vi "Update and Rename Files.vi"(8 "error in":errorcluster, 9 "Type ID":string="test", 10 "New Name":string="test", 11 "New PE Folder":path=path "C:/Users/carls/Desktop/test") -> (0 "error out":errorcluster)   [LabVIEW 2020, in "ADAS_IO_Template_MDO.lvclass"]
uses:
  ADAS_IO_Template_MDO.lvclass
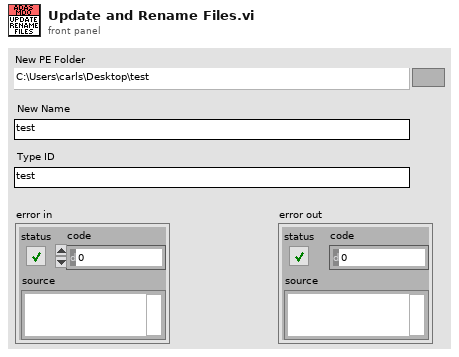
[diagram p1: front panel]
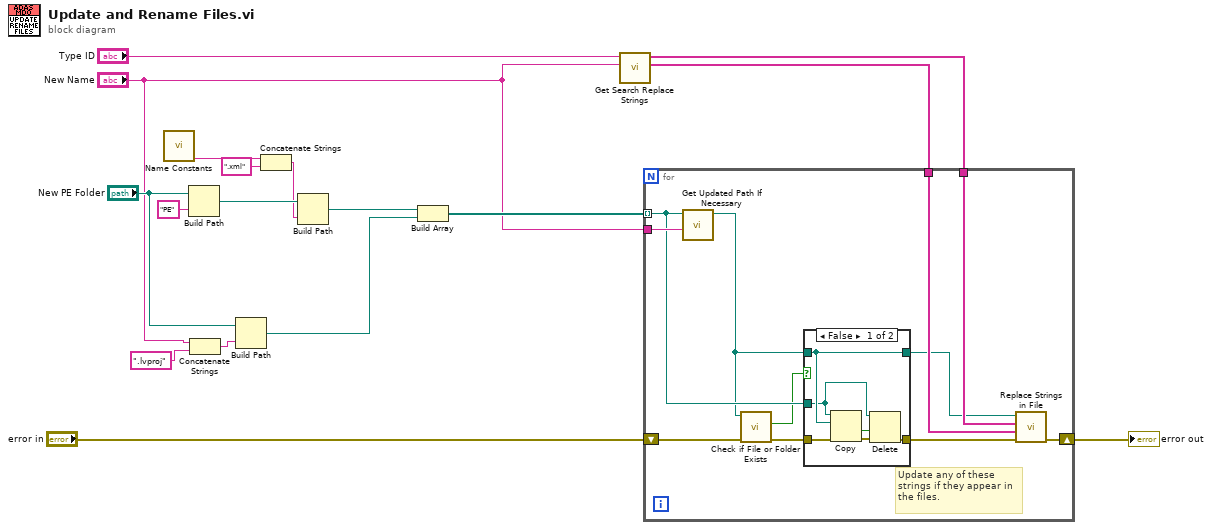
[diagram p0: block diagram]
diagram:
  n1 = call "Name Constants.vi"() -> ("Template Name"=w14:string)  [unwired: 9 in, 2 out]
  n2 = Build Path(base path="New PE Folder", name or relative path="PE") -> (appended path=w12:path)
  n3 = Concatenate Strings("New Name", ".lvproj" ("string")) -> (w1:string)
  n4 = Build Path(base path="New PE Folder", name or relative path=w1) -> (appended path=w8:path)
  n5 = Concatenate Strings(w14, ".xml" ("string")) -> (w11:string)
  n6 = Build Path(base path=w12, name or relative path=w11) -> (appended path=w10:path)
  n7 = Build Array(w10, w8) -> (w7:path[])
  n8 = call "Get Search Replace Strings.vi"("New Name"="New Name", "GUID"="Type ID") -> ("Replacement Strings"=w4:string[], "Search Strings"=w5:string[])  [unwired: 8 in]
  n9 = for {
    shift-right: [w28] -> w15
    shift-left: "error in" -> [w19]
    tunnel: w4 -> [w27]
    tunnel: w5 -> [w26]
    tunnel: "New Name" -> [w25]
    tunnel: w7 -> [w23] mode=indexing
    # "Update any of these\nstrings if they appear in\nthe files."
    n10 = call "Get Updated Path If Necessary.vi"("New Name"=w25, "Original Path"=w23) -> ("New Path"=w21:path)  [unwired: 8 in, 1 out]
    n11 = call <vilib>:"Check if File or Folder Exists.vi"("error in (no error)"=w19, "path"=w21) -> ("error out"=w18:errorcluster, "file or folder exists?"=w20:bool)  [unwired: 7 in, 1 out]
    n12 = case shown="False" w20 {
      tunnel: w21 -> [w32 w36]
      tunnel: [w32 w36] -> w24
      tunnel: w23 -> [w31 _]
      tunnel: w18 -> [w30 w35]
      tunnel: [w29 w35] -> w22
      frame False {
        n13 = Copy(8:w30, 10:w32, 11:w31) -> (0:w34:errorcluster, 1:w33:bool)  [unwired: 2 in, 1 out]
        n14 = Delete(path (use dialog)=w31, confirm (F)=w33, error in=w34) -> (error out=w29:errorcluster)  [unwired: 2 in, 2 out]
      }
      frame True {
      }
    }
    n15 = call "Replace Strings in File.vi"("error in"=w22, "Replace Strings"=w27, "Search Strings"=w26, "File Path"=w24) -> ("error out"=w28:errorcluster)  [unwired: 7 in]
  }
  "error out" <- w15
